vi "Set Greeter_req.vi"(7 "Complete Call (T)":bool=TRUE, 8 "error in (no error)":errorcluster, 10 "package_templatemessage":T1, 11 "gRPCid":T2) -> (0 "error out":errorcluster)   [LabVIEW 2019, in "Generated_server.lvlib"]
uses:
  Generated_server.lvlib
  <vilib>/gRPC/LabVIEW gRPC Library/Shared/grpcId.ctl
  Greeter_req.ctl
  Greeter_req_req_oneof/Greeter_req_req_oneof.lvclass
  Greeter_req_Flat.ctl
  Greeter_req_req_oneof/Greeter_req_req_oneof.lvclass/Greeter_req_req_oneof.ctl
  dcc74a39-081a-4bdd-860b-8ed792803c96.vi
  Greeter_req_req_oneof/GetActiveFieldIndex.vi
  Greeter_req_req_oneof/Getreq_int32.vi
  Greeter_req_req_oneof/Getreq_int64.vi
  Greeter_req_req_oneof/Getreq_uint32.vi
  Greeter_req_req_oneof/Getreq_uint64.vi
  Greeter_req_req_oneof/Getreq_sint32.vi
  Greeter_req_req_oneof/Getreq_sint64.vi
  Greeter_req_req_oneof/Getreq_fixed32.vi
  Greeter_req_req_oneof/Getreq_fixed64.vi
  Greeter_req_req_oneof/Getreq_sfixed32.vi
  Greeter_req_req_oneof/Getreq_sfixed64.vi
  Greeter_req_req_oneof/Getreq_float.vi
  Greeter_req_req_oneof/Getreq_double.vi
  Greeter_req_req_oneof/Getreq_bool.vi
  Greeter_req_req_oneof/Getreq_string.vi
  Greeter_req_req_oneof/Getreq_bytes.vi
  <vilib>/gRPC/LabVIEW gRPC Library/Shared/TranslateGrpcError.vi
  <vilib>/gRPC/LabVIEW gRPC Library/Server API/Server/Get Server DLL Path.vi
  <vilib>/Utility/error.llb/Error Cluster From Error Code.vi
  <vilib>/Utility/error.llb/Simple Error Handler.vi
  <vilib>/gRPC/LabVIEW gRPC Library/grpc-lvsupport-release.lvlib
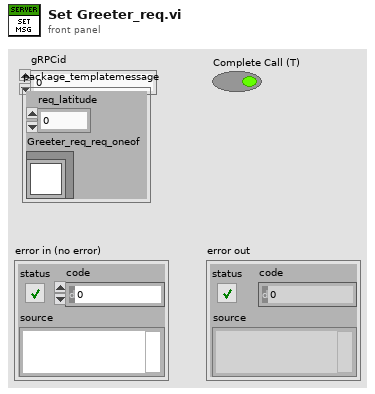
[diagram p1: front panel]
types:
  T1 = typedef "Generated_server.lvlib/Greeter_req.ctl" = cluster{"req_latitude":i32, "Greeter_req_req_oneof":refnum<class "Greeter_req_req_oneof.lvclass">}
  T2 = typedef "grpc-lvsupport-release.lvlib/grpcId.ctl" = u64
  T3 = typedef "Generated_server.lvlib/Greeter_req_Flat.ctl" = cluster{"req_latitude":i32, "Greeter_req_req_oneof_selected_index":i32, "req_int32":i32, "req_int64":i64, "req_uint32":u32, "req_uint64":u64, "req_sint32":i32, "req_sint64":i64, "req_fixed32":u32, "req_fixed64":u64, "req_sfixed32":i32, "req_sfixed64":i64, "req_float":sgl, "req_double":dbl, "req_bool":bool, "req_string":string, "req_bytes":u8[]}
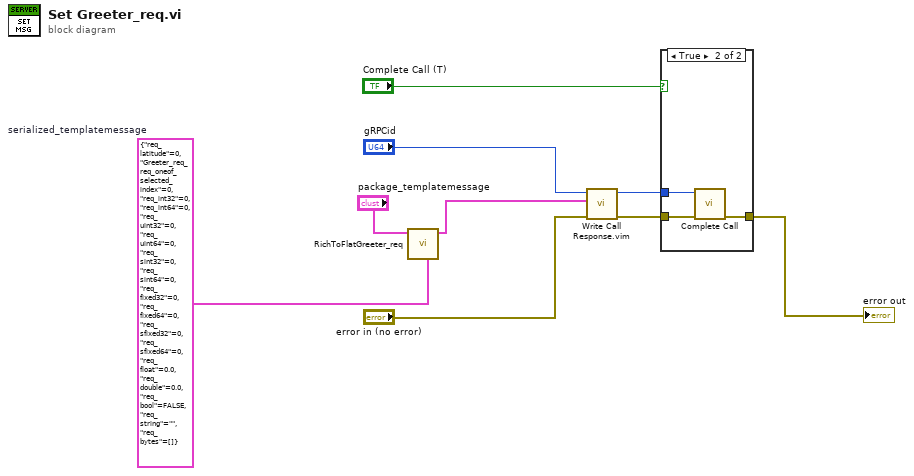
[diagram p0: block diagram]
diagram:
  w2 = T3 {"req_latitude"=0, "Greeter_req_req_oneof_selected_index"=0, "req_int32"=0, "req_int64"=0, "req_uint32"=0, "req_uint64"=0, "req_sint32"=0, "req_sint64"=0, "req_fixed32"=0, "req_fixed64"=0, "req_sfixed32"=0, "req_sfixed64"=0, "req_float"=0.0, "req_double"=0.0, "req_bool"=FALSE, "req_string"="", "req_bytes"=[]}  # serialized_templatemessage
  n1 = call "RichToFlatGreeter_req.vi"("OutputClusterType"=w2, "InputCluster"="package_templatemessage") -> ("OutputCluster"=w1:T3)  [unwired: 9 in]
  n2 = call "Write Call Response.vim"("error in"="error in (no error)", "Response Data"=w1, "gRPCid in"="gRPCid") -> ("error out"=w6:errorcluster, "gRPCid out"=w7:T2)  [unwired: 7 in]
  n3 = case shown="True" "Complete Call (T)" {
    tunnel: [w10 w13] -> w9
    tunnel: w7 -> [_ w12]
    tunnel: w6 -> [w10 w11]
    frame False {
    }
    frame True {
      n4 = call <vilib>:"Complete Call.vi"("gRPCid"=w12, "error in"=w11) -> ("error out"=w13:errorcluster)  [unwired: 8 in]
    }
  }
  "error out" <- w9
